vi "CreateVolumeScan.vi"(11 "Scan Settings":T1) -> (3 "Points":i16[][](array[numeric]))   [LabVIEW 2009]
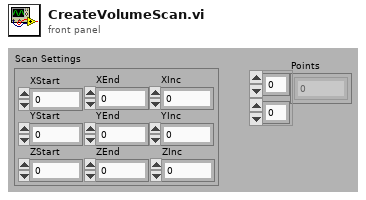
[diagram p1: front panel]
types:
  T1 = cluster{"XStart":i16, "XEnd":i16, "XInc":i16, "YStart":i16, "YEnd":i16, "YInc":i16, "ZStart":i16, "ZEnd":i16, "ZInc":i16}
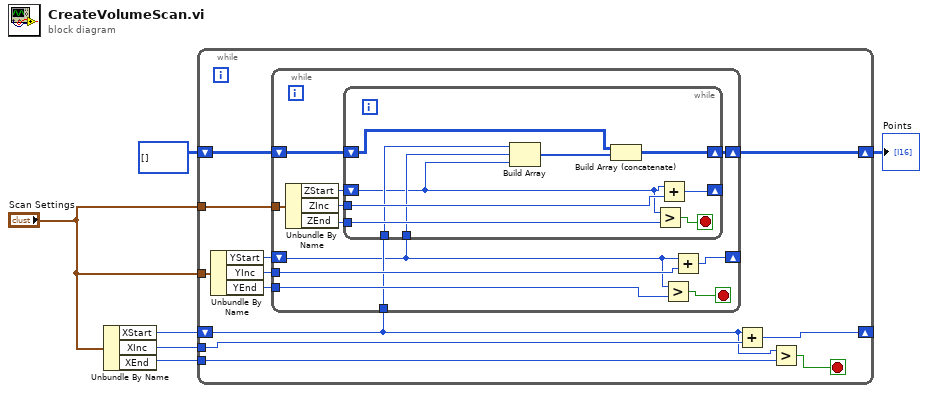
[diagram p0: block diagram]
diagram:
  n1 = Unbundle By Name("Scan Settings") -> ("XStart"=w6:i16, "XInc"=w5:i16, "XEnd"=w4:i16)
  n2 = while {
    shift-right: [w17] -> _
    shift-left: w6 -> [w9]
    tunnel: w5 -> [w18]
    tunnel: w4 -> [w16]
    tunnel: "Scan Settings" -> [w14]
    tunnel: "Scan Settings" -> [w10]
    shift-right: [w8] -> w1
    shift-left: i16[][] [] -> [w7]
    stop <- w15 stop-if-true
    n3 = Unbundle By Name(w14) -> ("YStart"=w13:i16, "YInc"=w12:i16, "YEnd"=w11:i16)
    n4 = while {
      shift-right: [w30] -> _
      shift-left: w13 -> [w21]
      tunnel: w12 -> [w29]
      tunnel: w11 -> [w27]
      tunnel: w10 -> [w26]
      tunnel: w9 -> [w22]
      shift-right: [w20] -> w8
      shift-left: w7 -> [w19]
      stop <- w28 stop-if-true
      n5 = Unbundle By Name(w26) -> ("ZStart"=w25:i16, "ZInc"=w24:i16, "ZEnd"=w23:i16)
      n6 = while {
        shift-right: [w40] -> _
        shift-left: w25 -> [w34]
        tunnel: w24 -> [w39]
        tunnel: w23 -> [w37]
        tunnel: w22 -> [w36]
        tunnel: w21 -> [w35]
        shift-right: [w32] -> w20
        shift-left: w19 -> [w31]
        stop <- w38 stop-if-true
        n7 = Build Array(w36, w35, w34) -> (w33:i16[])
        n8 = Build Array (concatenate)(w31, w33) -> (w32:i16[][])
        n9 = Greater?(x=w34, y=w37) -> (0:w38:bool)
        n10 = Add(x=w34, y=w39) -> (x+y=w40:i16)
      }
      n11 = Greater?(x=w21, y=w27) -> (0:w28:bool)
      n12 = Add(x=w21, y=w29) -> (x+y=w30:i16)
    }
    n13 = Add(x=w9, y=w18) -> (x+y=w17:i16)
    n14 = Greater?(x=w9, y=w16) -> (0:w15:bool)
  }
  "Points" <- w1
